vi "Error logger.vi"(8 "error IO":errorcluster, 11 "ER":refnum<queue>) -> ()   [LabVIEW 2022 SP3]
panel:
  out "error out":errorcluster
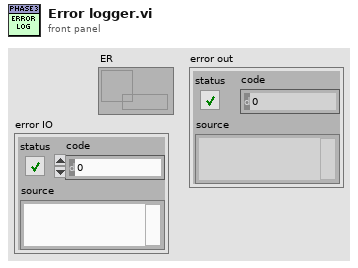
[diagram p1: front panel]
types:
  T1 = enum16{"Initialise", "Poll Event", "Logg Error", "Exit"}
  T2 = enum16{"open", "replace", "create", "open or create", "replace or create", "replace or create with confirmation"}
  T3 = cluster{"Info  Folder path":path, " Ground Systems Data Log Folder Path ":path, "RT  Error log Folder Path":path, "Login Details  Folder Path":path, "HW Configaration  Folder Path":path, "Signal Folder Path":path, "Test Settings Data Log Folder Path ":path, "System Setting Sequence Folder Path":path, "Sequence Folder Path":path, "Sub VI's  Folder Path":path, "DAQ  VI's  Folder Path":path, "Source Code  Folder Path":path, "Log In Module  Folder Path ":path, "Button Operations Folder Path":path, "Vehicle Data transmitter Log Folder Path ":path, "Vehicle Data Receiver Log Folder Path ":path, "ec_download_path":path, "ec_upload_path":path, "fc_upload_path":path, "fc_download_path":path, "Avionics File Path ":path, "Fault Data":path, "MCRC Error log Folder Path":path, "USB File Transfer Path":path}
  T4 = cluster{"Error Code":string, "Error Source":string}
  T5 = cluster{"Start DAQ":bool, "Stop DAQ":bool, "Start DataLog":bool, "Stop Datalog":bool, "Restart Datalog ":bool, "Exit":bool, "Datalog Title":string, "LCC IP Address:":string}
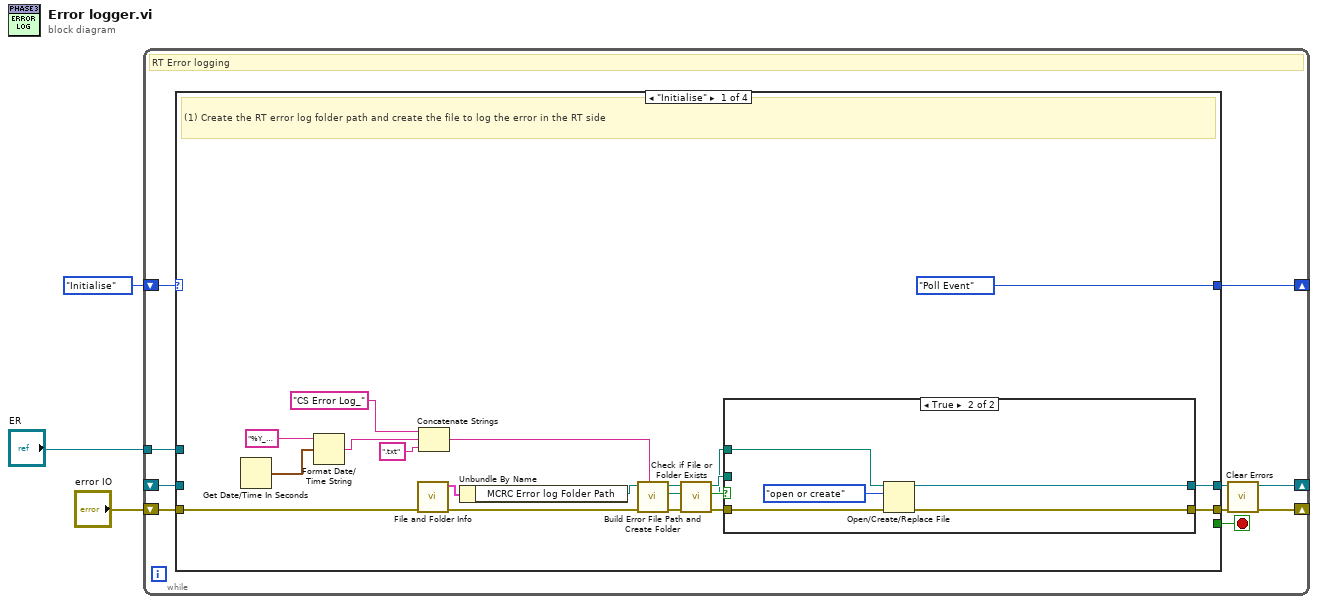
[diagram p0: block diagram]
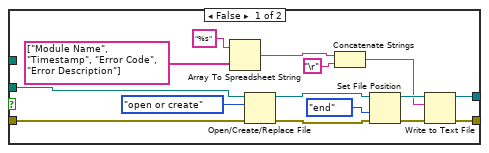
[diagram p2: hidden frame]
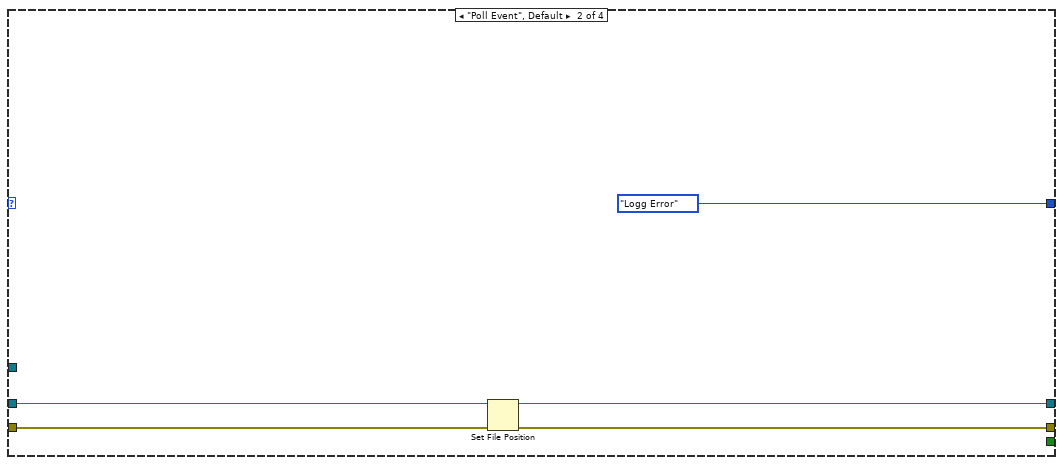
[diagram p3: hidden frame]
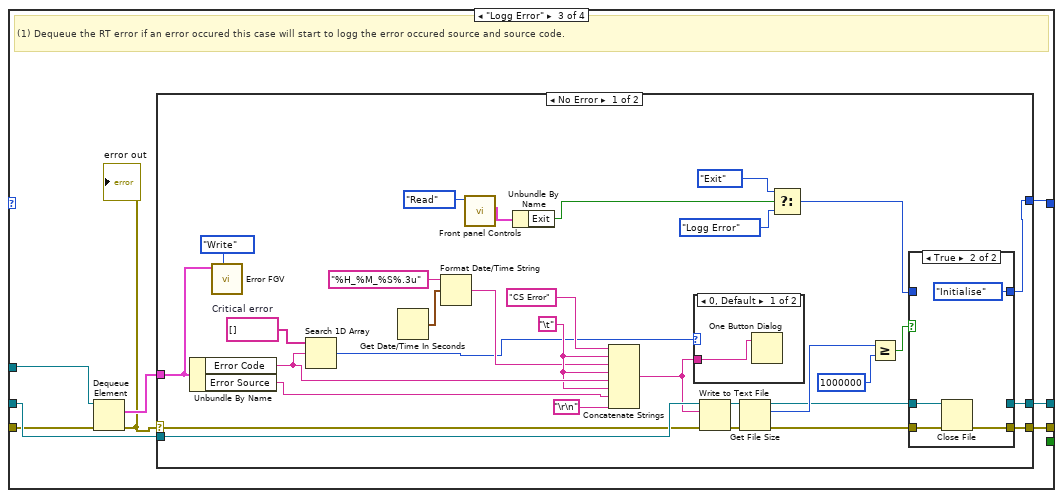
[diagram p4: hidden frame]
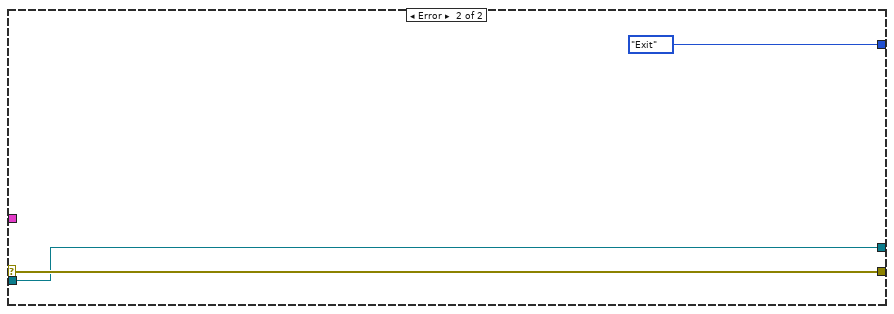
[diagram p7: hidden frame]
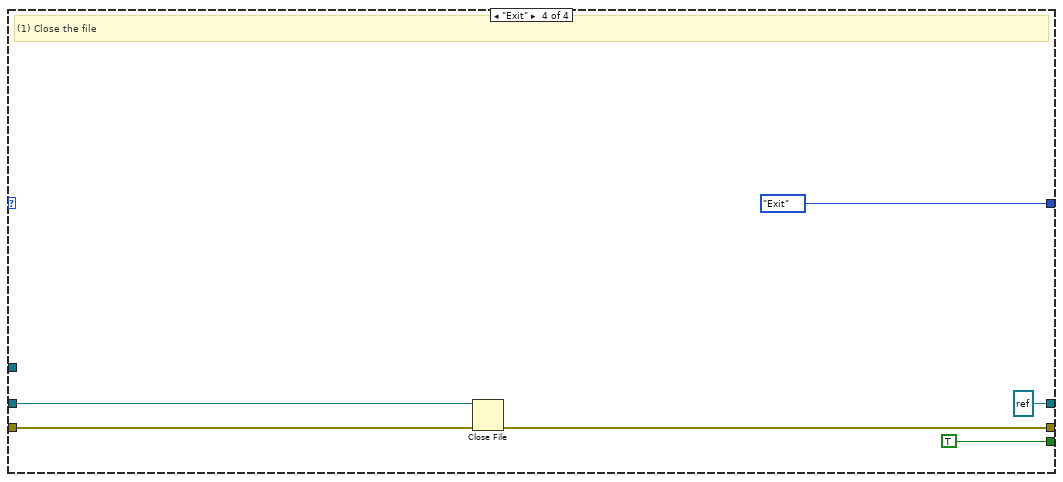
[diagram p8: hidden frame]
diagram:
  n1 = while {
    shift-right: [w11] -> _
    shift-left: T1."Initialise" -> [w12]
    shift-right: [w10] -> _
    shift-left: _ -> [w9]
    shift-right: [w4] -> _
    shift-left: "error IO" -> [w8]
    tunnel: "ER" -> [w5]
    stop <- w6 stop-if-true
    # "RT Error logging"
    n2 = case shown="\"Initialise\"" w12 {
      tunnel: [T1."Poll Event" T1."Logg Error" w58 T1."Exit"] -> w11
      tunnel: [w23 w55 w62 refnum<file> refnum ("refnum out")] -> w10
      tunnel: w9 -> [_ w56 w63 w110]
      tunnel: w8 -> [w20 w54 w60 w109]
      tunnel: [w21 w53 w61 w108] -> w7
      tunnel: [_ _ _ TRUE] -> w6
      tunnel: w5 -> [_ _ w57 _]
      frame "Initialise" {
        # "(1) Create the RT error log folder path and create the file to log the error in the RT side"
        n3 = Get Date/Time In Seconds() -> (seconds since 1Jan1904=w16:timestamp)
        n4 = Format Date/Time String(time format string (%c)="%Y_%b_%d_%Hh_%Mm_%Ssec", seconds (now)=w16) -> (date/time string=w15:string)  [unwired: 1 in]
        n5 = call "File and Folder Info.vi"("error in (no error)"=w20) -> ("error out"=w30:errorcluster, "Path Cluster 2"=w31:T3)  [unwired: 9 in]
        n6 = Concatenate Strings("CS Error Log_" ("string"), w15, ".txt" ("string")) -> (w13:string)
        n7 = Unbundle By Name(w31) -> ("MCRC Error log Folder Path"=w14:path)
        n8 = call "Build Error File Path and Create Folder.vi"("File Name"=w13, "error in (no error)"=w30, "Base Path"=w14) -> ("error out"=w28:errorcluster, "Result File path"=w18:path, "Result Folder path"=w29:path)  [unwired: 6 in]
        n9 = call <vilib>:"Check if File or Folder Exists.vi"("error in (no error)"=w28, "path"=w29) -> ("error out"=w22:errorcluster, "file or folder exists?"=w24:bool, "dup path"=w19:path)  [unwired: 7 in]
        n10 = case shown="True" w24 {
          tunnel: [w42 w50] -> w23
          tunnel: w22 -> [w45 w49]
          tunnel: [w41 w48] -> w21
          tunnel: w19 -> [w32 _]
          tunnel: w18 -> [_ w47]
          frame False {
            n11 = Array To Spreadsheet String(array=string[] ["Module Name", "Timestamp", "Error Code", "Error Description"], 3:"%s" ("format string")) -> (spreadsheet string=w36:string)  [unwired: 1 in]
            n12 = Open/Create/Replace File(file path (use dialog)=w32, error in=w45, operation (0:open)=T2."open or create") -> (refnum out=w44:refnum<file>, error out=w43:errorcluster)  [unwired: 3 in, 1 out]
            n13 = Concatenate Strings(w36, "\r") -> (w34:string)
            n14 = Set File Position(refnum=w44, from (0:start)=enum16{"start", "end", "current"}."end", error in=w43) -> (refnum out=w40:refnum<file>, error out=w39:errorcluster)  [unwired: 1 in]
            n15 = Write to Text File(file (use dialog)=w40, text=w34, error in=w39) -> (refnum out=w42:refnum<file>, error out=w41:errorcluster)  [unwired: 1 in, 1 out]
          }
          frame True {
            n16 = Open/Create/Replace File(file path (use dialog)=w47, error in=w49, operation (0:open)=T2."open or create") -> (refnum out=w50:refnum<file>, error out=w48:errorcluster)  [unwired: 3 in, 1 out]
          }
        }
      }
      frame "Poll Event", Default {
        n17 = Set File Position(refnum=w56, error in=w54) -> (refnum out=w55:refnum<file>, error out=w53:errorcluster)  [unwired: 2 in]
      }
      frame "Logg Error" {
        # "(1) Dequeue the RT error if an error occured this case will start to logg the error occured source and source code."
        n18 = Dequeue Element(queue=w57, error in (no error)=w60) -> (element=w64:T4, error out=w59:errorcluster)  [unwired: 1 in, 2 out]
        "error out" <- w59
        n19 = case shown="No Error" w59 {
          selector: w59 -> [w86 w106]
          tunnel: w64 -> [w71 _]
          tunnel: w63 -> [w95 w105]
          tunnel: [w76 w105] -> w62
          tunnel: [w78 w106] -> w61
          tunnel: [w75 T1."Exit"] -> w58
          frame No Error {
            w88 = string[] []  # Critical error
            w91 = "\t"
            n20 = Unbundle By Name(w71) -> ("Error Code"=w94:string, "Error Source"=w93:string)
            n21 = call "Error FGV.vi"("Enum"=enum16{"Read", "Write", "Clear"}."Write", "CS err"=w71) -> ()  [unwired: 9 in, 1 out]
            n22 = Search 1D Array(1D array=w88, element=w94) -> (index of element=w87:i32)  [unwired: 1 in]
            n23 = Get Date/Time In Seconds() -> (seconds since 1Jan1904=w68:timestamp)
            n24 = Format Date/Time String(time format string (%c)="%H_%M_%S%.3u", seconds (now)=w68) -> (date/time string=w90:string)  [unwired: 1 in]
            n25 = call "Front panel Controls.vi"("Write/Read"=enum16{"Write", "Read"}."Read") -> ("Front Panel Control (R)"=w67:T5)  [unwired: 9 in, 1 out]
            n26 = Unbundle By Name(w67) -> ("Exit"=w65:bool)
            n27 = Concatenate Strings("CS Error" ("string"), w91, w90, w91, w94, w91, w93, "\r\n") -> (w73:string)
            n28 = case shown="0, Default" w87 {
              tunnel: w73 -> [w103 _]
              frame 0, Default {
                n29 = One Button Dialog(message=w103) -> ()  [unwired: 1 in, 1 out]
              }
              frame -1 {
              }
            }
            n30 = Write to Text File(file (use dialog)=w95, text=w73, error in=w86) -> (refnum out=w83:refnum<file>, error out=w84:errorcluster)  [unwired: 1 in, 1 out]
            n31 = Get File Size(file=w83, error in=w84) -> (refnum out=w77:refnum<file>, size (in bytes)=w82:i64, 0:w79:errorcluster)
            n32 = Select(t=T1."Exit", s=w65, f=T1."Logg Error") -> (s? t:f=w74:T1)
            n33 = Greater Or Equal?(x=w82, y=i64 1000000) -> (x >= y?=w80:bool)
            n34 = case shown="True" w80 {
              tunnel: w79 -> [w98 w100]
              tunnel: [w98 w101] -> w78
              tunnel: w77 -> [w97 w102]
              tunnel: [w97 _] -> w76
              tunnel: [w96 T1."Initialise"] -> w75
              tunnel: w74 -> [w96 _]
              frame False {
              }
              frame True {
                n35 = Close File(refnum=w102, error in=w100) -> (error out=w101:errorcluster)  [unwired: 1 out]
              }
            }
          }
          frame Error {
          }
        }
      }
      frame "Exit" {
        # "(1) Close the file"
        n36 = Close File(refnum=w110, error in=w109) -> (error out=w108:errorcluster)  [unwired: 1 out]
      }
    }
    n37 = call <vilib>:"Clear Errors.vi"("error in (no error)"=w7) -> ("error out"=w4:errorcluster)  [unwired: 5 in, 1 out]
  }
